vi "Remove Alias.vi"(8 "error in (no error)":errorcluster, 10 "Alias":string, 11 "Aliases Section Ptr in":T1 format="%.0x") -> (0 "error out":errorcluster, 1 "Removed":bool, 3 "Aliases Section Ptr out":T1 format="%.0x")   [LabVIEW 2017, in "Switch Scripting.lvlib"]
uses:
  Switch Scripting.lvlib
  <vilib>/NI Veristand/Custom Device API/Custom Device Item Ref.ctl
  <vilib>/NI VeriStand/Custom Device API/Custom Device API.lvlib
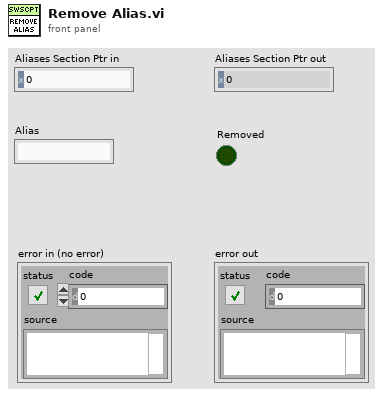
[diagram p1: front panel]
types:
  T1 = typedef "Custom Device API.lvlib/Custom Device Item Ref.ctl" = u64
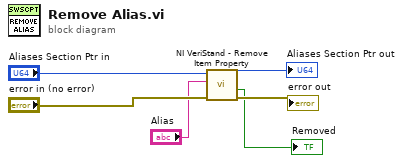
[diagram p0: block diagram]
diagram:
  n1 = call <vilib>:"NI VeriStand - Remove Item Property.vi"("error in (no error)"="error in (no error)", "Property Name"="Alias", "Item Ref in"="Aliases Section Ptr in") -> ("error out"=→"error out":errorcluster, "Removed"=→"Removed":bool, "Item Ref out"=→"Aliases Section Ptr out":T1)  [unwired: 6 in]
